vi "Config path--constant.vi"(8 "error in (no error)":errorcluster) -> (0 "error out":errorcluster, 3 "Config Path":path)   [LabVIEW 2019, in "Panther Dashboard.lvlib"]
uses:
  Panther Dashboard.lvlib
  <vilib>/Utility/sysdir.llb/System Directory Type.ctl
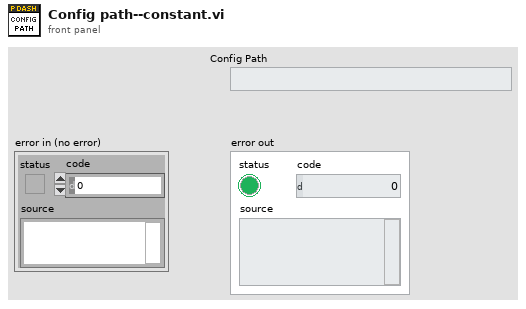
[diagram p1: front panel]
types:
  T1 = typedef "System Directory Type.ctl" = i32
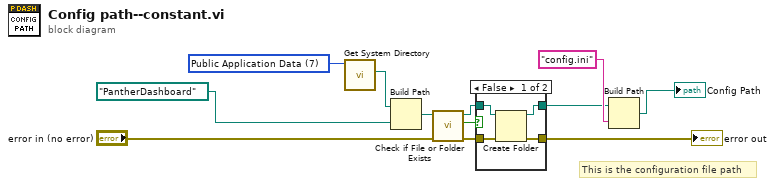
[diagram p0: block diagram]
diagram:
  w9 = T1 7 items=["User Home"=0, "User Desktop"=1, "User Documents"=2, "User Application Data"=3, "User Preferences"=4, "User Temporary"=5, "Public Documents"=6, "Public Application Data"=7, "Public Preferences"=8, "Public Cache"=13, "System Core Libraries"=9, "System Installed Libraries"=10, "Application Files"=11, "Boot Volume Root"=12] ("system directory type")
  # "This is the configuration file path"
  n1 = call <vilib>:"Get System Directory.vi"("system directory type"=w9) -> ("system directory"=w8:path)  [unwired: 10 in]
  n2 = Build Path(base path=w8, name or relative path=path "PantherDashboard") -> (appended path=w2:path)
  n3 = call <vilib>:"Check if File or Folder Exists.vi"("error in (no error)"="error in (no error)", "path"=w2) -> ("error out"=w12:errorcluster, "file or folder exists?"=w3:bool, "dup path"=w4:path)  [unwired: 7 in]
  n4 = case shown="False" w3 {
    tunnel: [w13 w17] -> w5
    tunnel: w4 -> [w14 w17]
    tunnel: w12 -> [w16 w18]
    tunnel: [w15 w18] -> w11
    frame False {
      n5 = Create Folder(path (use dialog)=w14, error in=w16) -> (created path=w13:path, error out=w15:errorcluster)  [unwired: 1 in, 1 out]
    }
    frame True {
    }
  }
  "error out" <- w11
  n6 = Build Path(base path=w5, name or relative path="config.ini") -> (appended path=→"Config Path":path)
